vi "TP Buffer Search for Connection.vi"(0 "Connecctions":T3[](array[typedef]), 5 "CAN frame":T1 {"payload" format="%x"; "timestamp" format="%<%.7X\n%x>T"; "type" items=["CAN Data"=0, "CAN Remote"=1, "CAN Bus Error"=2, "Delay"=224, "Log Trigger"=225, "Start Trigger"=226]; "identifier" format="%x"}, 11 "error in (no error)":errorcluster) -> (4 "Connection Cluster Out":T3, 6 "CAN frame Out":T1 {"payload" format="%x"; "timestamp" format="%<%.7X\n%x>T"; "type" items=["CAN Data"=0, "CAN Remote"=1, "CAN Bus Error"=2, "Delay"=224, "Log Trigger"=225, "Start Trigger"=226]; "identifier" format="%x"}, 8 "Found?":bool, 10 "Index":i32, 15 "error out":errorcluster)   [LabVIEW 2013, in "J1939 Addon Engine.lvlib"]
uses:
  Engine/J1939 Addon Engine.lvlib
  Types/TP Buffer Connection Cluster.ctl
  <vilib>/xnet/xnet.llb/XNET Frame CAN.ctl
  <vilib>/xnet/xnet.llb/XNET Frame Type CAN.ctl
  J1939 Utilities/SubVIs/Convert CAN Arb ID to J1939 ID.vi
  J1939 Utilities/J1939 Utilities.lvlib
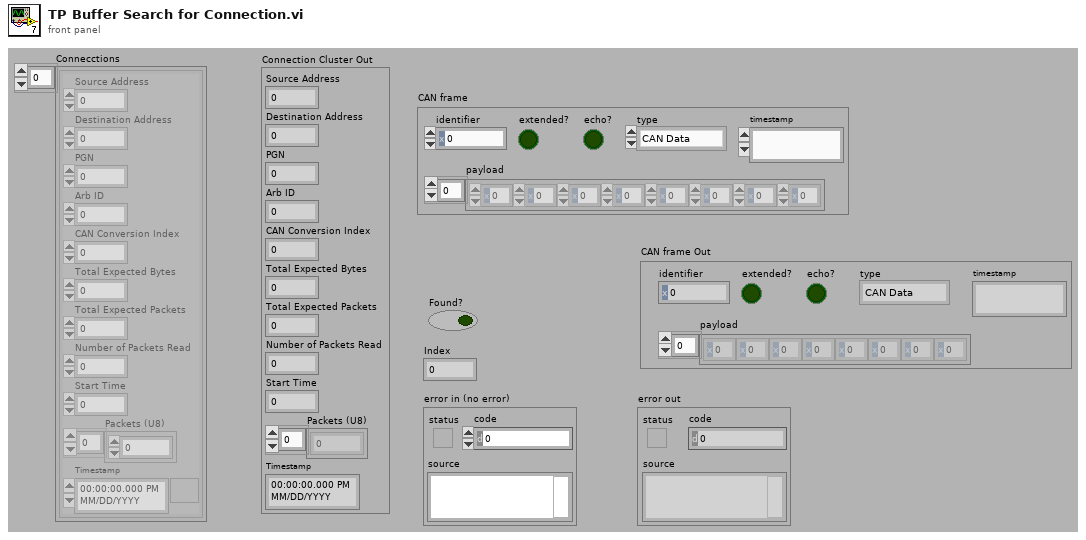
[diagram p1: front panel]
types:
  T1 = typedef "XNET Frame CAN.ctl" = cluster{"timestamp":timestamp, "payload":u8[], "identifier":u32, "type":T2, "extended?":bool, "echo?":bool}
  T2 = typedef "XNET Frame Type CAN.ctl" = u8
  T3 = typedef "J1939 Addon Engine.lvlib/TP Buffer Connection Cluster.ctl" = cluster{"Source Address":u8, "Destination Address":u8, "PGN":u32, "Arb ID":u32, "CAN Conversion Index":u32, "Total Expected Bytes":u16, "Total Expected Packets":u8, "Number of Packets Read":u8, "Start Time":u32, "Packets (U8)":u8[], "Timestamp":timestamp}
  T4 = typedef "J1939 Utilities.lvlib/PGN Fields Cluster.ctl" = cluster{"Reserved Bit":u8, "Data page":u8, "PDU Format":u8, "PDU Specific":u8}
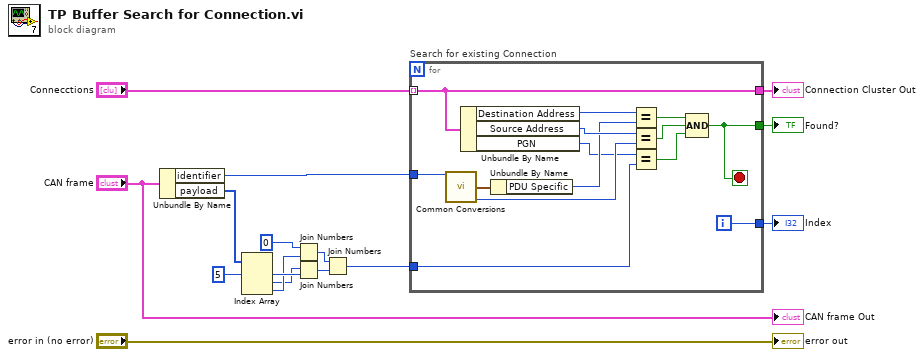
[diagram p0: block diagram]
diagram:
  n1 = Unbundle By Name("CAN frame") -> ("identifier"=w12:u32, "payload"=w2:u8[])
  n2 = Index Array(array=w2, index #1=5 ("index")) -> (element #1=w9:u8, element #2=w4:u8, element #3=w8:u8)  [unwired: 2 in]
  n3 = Join Numbers(hi=u8 0, lo=w8) -> ((hi.lo)=w5:u16)
  n4 = Join Numbers(hi=w4, lo=w9) -> ((hi.lo)=w6:u16)
  n5 = Join Numbers(hi=w5, lo=w6) -> ((hi.lo)=w1:u32)
  n6 = for "Search for existing Connection" {
    tunnel: "Connecctions" -> [w21] mode=indexing
    tunnel: w12 -> [w28]
    tunnel: [w22] -> w16
    tunnel: [w21] -> w14
    tunnel: [w20] -> w13
    tunnel: w1 -> [w18]
    i -> [w20]
    stop <- w22 stop-if-true
    n7 = call-poly "Common Conversions.vi"("Arb ID"=w28) -> ("PGN Fields"=w29:T4, "Source Address"=w26:u8)  [unwired: 13 out]
    n8 = Unbundle By Name(w21) -> ("Destination Address"=w30:u8, "Source Address"=w27:u8, "PGN"=w19:u32)
    n9 = Unbundle By Name(w29) -> ("PDU Specific"=w25:u8)
    n10 = Equal?(x=w30, y=w25) -> (x = y?=w24:bool)
    n11 = Equal?(x=w27, y=w26) -> (x = y?=w23:bool)
    n12 = Equal?(x=w19, y=w18) -> (x = y?=w17:bool)
    n13 = Compound Arithmetic op=AND(w24, w23, w17) -> (w22:bool)
  }
  "Found?" <- w16
  "Connection Cluster Out" <- w14
  "Index" <- w13
  "error out" <- "error in (no error)"
  "CAN frame Out" <- "CAN frame"
